vi "Actor core.vi"(8 "error in (no error)":errorcluster, 11 "Cap Bank Server in":refnum<class "Cap Bank Server.lvclass">) -> (0 "error out":errorcluster, 3 "Actor out":refnum<class "Actor.lvclass">)   [LabVIEW 2015, in "Cap Bank Server.lvclass"]
uses:
  Cap Bank Server/Cap Bank Server.lvclass
  <vilib>/ActorFramework/Actor/Actor.lvclass
  <vilib>/ActorFramework/Actor/Actor.lvclass/Actor.ctl
  <vilib>/ActorFramework/Message Enqueuer/Message Enqueuer.lvclass/Message Enqueuer.ctl
  Cap Bank Server/Cap Bank Server.lvclass/Cap Bank Server.ctl
  <vilib>/ActorFramework/Message Enqueuer/Init from Existing Queue.vi
  <vilib>/ActorFramework/Message Enqueuer/Enqueue.vi
  <vilib>/ActorFramework/Message Priority Queue/Priority Enqueue.vi
  Mag Lab Measure Controller.lvclass
  <vilib>/ActorFramework/Message Enqueuer/Message Enqueuer.lvclass
  Cap Bank Server Messages/Update plot from list Msg/Update plot from list Msg.lvclass
  <vilib>/ActorFramework/Stop Msg/Stop Msg.lvclass
panel:
  in  "Magnet pulses":i32(listbox)
  out "Shot data":string
  out "Idot Graph":waveform(dbl)[](graph)
  out "Log":string
  in  "stop":bool
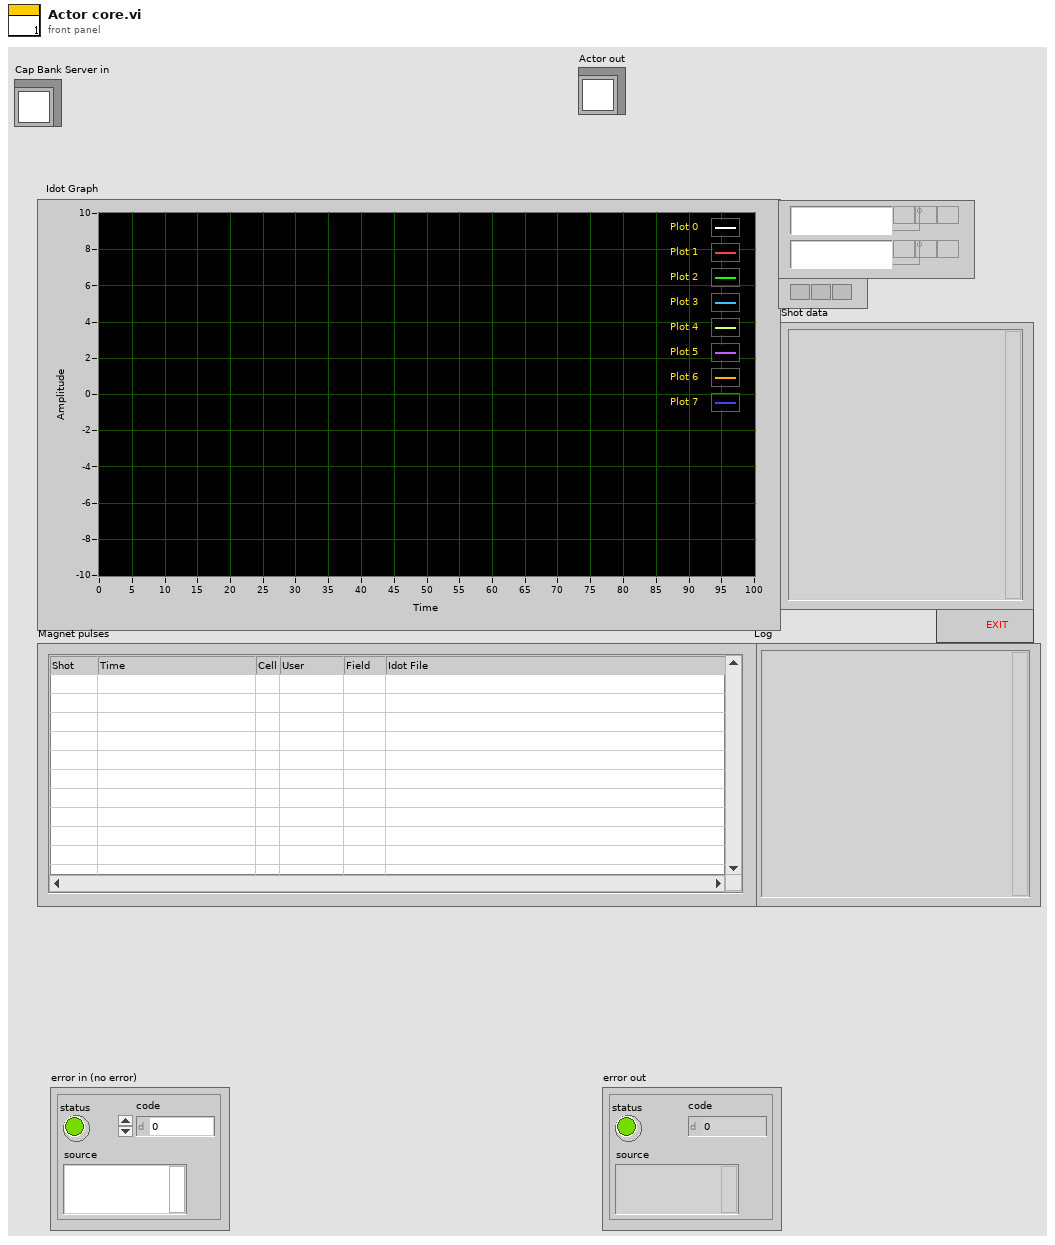
[diagram p1: front panel]
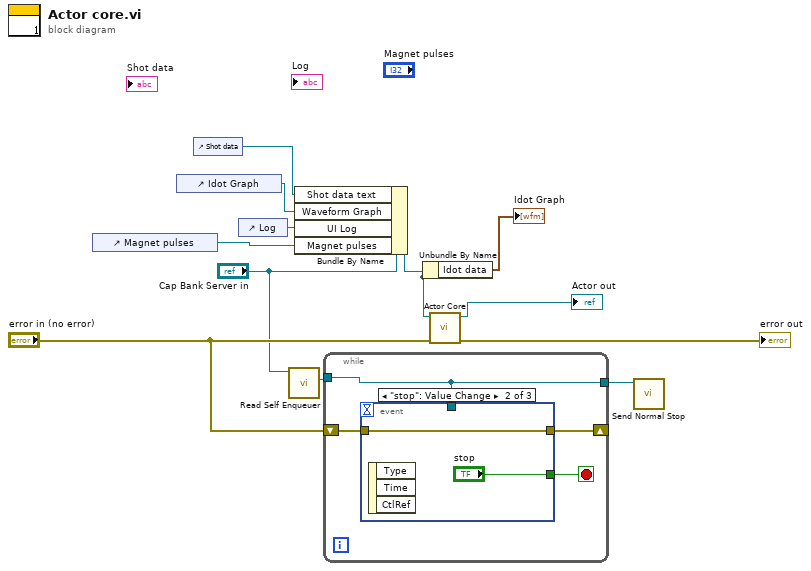
[diagram p0: block diagram]
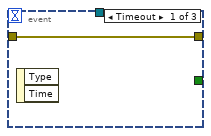
[diagram p2: hidden frame]
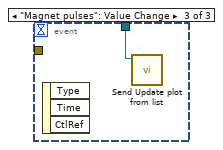
[diagram p3: hidden frame]
diagram:
  n1 = control-ref of="Magnet pulses"() -> (w1:refnum<vi>)
  n2 = control-ref of="Idot Graph"() -> (w3:refnum<vi>)
  n3 = control-ref of="Shot data"() -> (w2:refnum<vi>)
  n4 = control-ref of="Log"() -> (w7:refnum<vi>)
  n5 = call <vilib>:"Read Self Enqueuer.vi"("Actor"="Cap Bank Server in") -> ("Self Enqueuer"=w9:refnum<class "Message Enqueuer.lvclass">)  [unwired: 10 in]
  n6 = Bundle By Name(cluster="Cap Bank Server in", "Shot data text"=w2, "Waveform Graph"=w3, "UI Log"=w7, "Magnet pulses"=w1) -> (w5:refnum<class "Cap Bank Server.lvclass">)
  n7 = while {
    shift-right: [w14] -> _
    shift-left: "error in (no error)" -> [w15]
    tunnel: w9 -> [w13]
    tunnel: [w13] -> w8
    stop <- w16 stop-if-true
    n8 = event shown="[1] \"stop\": Value Change" {
      selector: _ -> [_ _ _]
      dyn-events: _ -> [_ _ _]
      timeout: _ -> [_ _ _]
      tunnel: [_ "stop" _] -> w16
      tunnel: w15 -> [w17 w18 _]
      tunnel: [w17 w18 _] -> w14
      tunnel: w13 -> [_ _ w20]
      event Timeout {
        n9 = event-data() -> ()  [unwired: 1 in, 2 out]
      }
      event "stop": Value Change {
        n10 = event-data() -> ()  [unwired: 1 in, 3 out]
      }
      event "Magnet pulses": Value Change {
        n11 = event-data() -> ()  [unwired: 1 in, 3 out]
        n12 = call "Send Update plot from list.vi"("Message Enqueuer"=w20) -> ()  [unwired: 9 in, 2 out]
      }
    }
  }
  n13 = Unbundle By Name(w5) -> ("Idot data"=→"Idot Graph":waveform(dbl)[])
  n14 = call-parent "Actor Core.vi"("error in"="error in (no error)", "Mag Lab Measure Base in"=w5) -> ("error out"=→"error out":errorcluster, "Actor out"=→"Actor out":refnum<class "Actor.lvclass">)  [unwired: 8 in]
  n15 = call <vilib>:"Send Normal Stop.vi"("Message Enqueuer"=w8) -> ()  [unwired: 10 in, 1 out]
